vi "DN4_ToErrorCluster_Polymorphic.vi"(3 "task id":i32=-1, 4 "error code":i32 format="%x") -> (1 "error out":errorcluster)   [LabVIEW 2020]
doc: "Translate DAQNavi's error code to labview's error cluster"
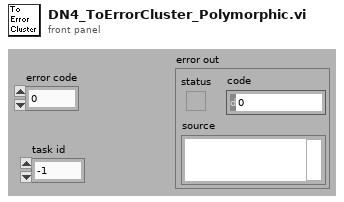
[diagram p1: front panel]
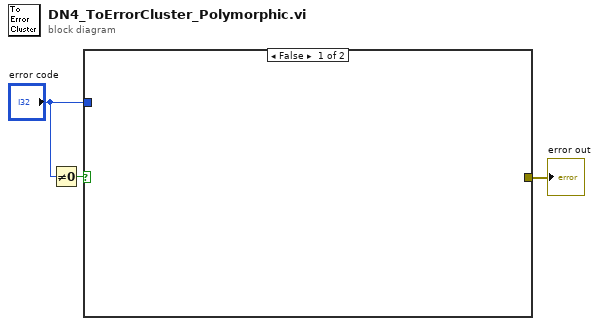
[diagram p0: block diagram]
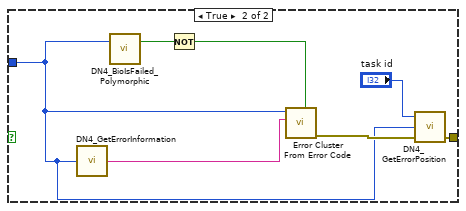
[diagram p2: hidden frame]
diagram:
  n1 = Not Equal To 0?(x="error code") -> (x != 0?=w2:bool)
  n2 = case shown="False" w2 {
    tunnel: [_ w8] -> w3
    tunnel: "error code" -> [_ w4]
    frame False {
    }
    frame True {
      n3 = call "DN4_GetErrorInformation.vi"("error code"=w4) -> ("info"=w10:string)
      n4 = call "DN4_BioIsFailed_Polymorphic.vi"("ErrorCode"=w4) -> ("IsFailed?"=w9:bool)  [unwired: 2 out]
      n5 = Not(x=w9) -> (.not. x?=w5:bool)
      n6 = call <vilib>:"Error Cluster From Error Code.vi"("is warning? (False)"=w5, "error message (\"\")"=w10, "error code (0)"=w4) -> ("error out"=w6:errorcluster)  [unwired: 2 in, 4 out]
      n7 = call "DN4_GetErrorPosition.vi"("error in (no error)"=w6, "error code"=w4, "task in"="task id") -> ("error out"=w8:errorcluster)  [unwired: 2 out]
    }
  }
  "error out" <- w3
